vi "EnQ Vacuum State.vi"(6 "Raw Pressure":dbl=nan, 7 "d/dt":dbl, 8 "error in (no error)":errorcluster, 9 "Pressure":dbl=nan, 10 "State":T1, 11 "cRIO Vacuum in":refnum<class "cRIO Vacuum.lvclass">) -> (0 "error out":errorcluster, 1 "overflow?":bool, 2 "Overflow State":T1, 3 "cRIO Vacuum out":refnum<class "cRIO Vacuum.lvclass">, 4 "Overflow Pressure":dbl, 5 "Overflow Raw Pressure":dbl)   [LabVIEW 2015, in "cRIO-Carbondioxide.lvlib" / "CO2-Actor.lvlib" / "cRIO Vacuum.lvclass"]
uses:
  cRIO Vacuum.lvclass
  Controls/Vacuum State Enumerator.ctl
  Controls/Vacuum State Cluster.ctl
  cRIO Vacuum.lvclass/cRIO Vacuum.ctl
panel:
  out "Overflow d/dt":dbl
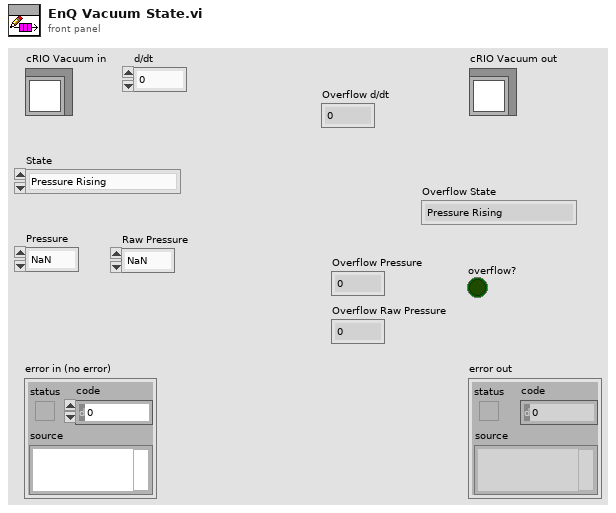
[diagram p1: front panel]
types:
  T1 = typedef "Vacuum State Enumerator.ctl" = enum16{"Pressure Rising", "Plateau", "Pressure Dropping", "Valley", "Low Valley", "Leak", "Unknown"}
  T2 = typedef "Vacuum State Cluster.ctl" = cluster{"Vacuum State":T1, "Pressure":dbl, "Raw Pressure":dbl, "d/dt":dbl}
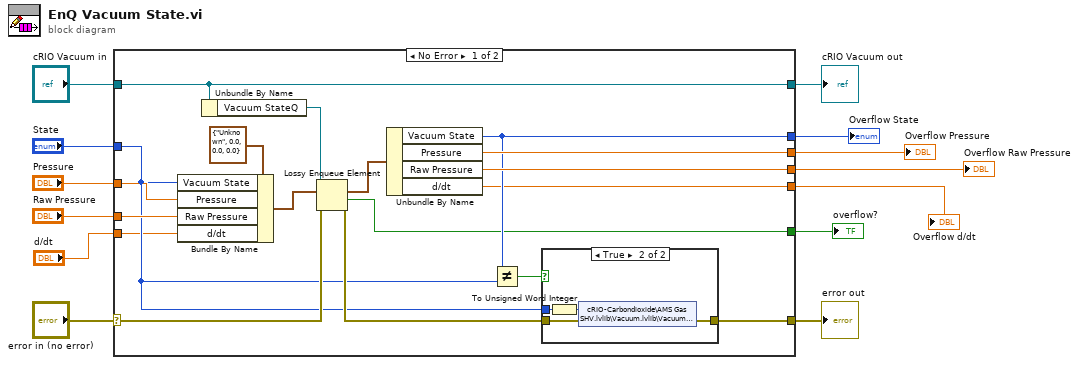
[diagram p0: block diagram]
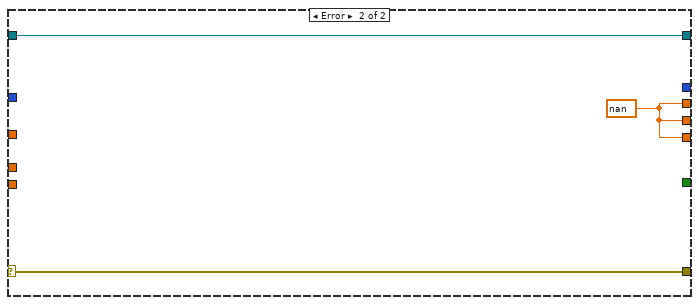
[diagram p3: hidden frame]
diagram:
  n1 = case shown="No Error" "error in (no error)" {
    selector: "error in (no error)" -> [w30 w38]
    tunnel: [w22 w38] -> w12
    tunnel: [w31 w39] -> w10
    tunnel: "cRIO Vacuum in" -> [w31 w39]
    tunnel: "State" -> [w20 _]
    tunnel: [w24 _] -> w8
    tunnel: [w15 _] -> w7
    tunnel: "Pressure" -> [w26 _]
    tunnel: [w28 w37] -> w5
    tunnel: "Raw Pressure" -> [w27 _]
    tunnel: [w25 w37] -> w3
    tunnel: "d/dt" -> [w16 _]
    tunnel: [w14 w37] -> w1
    frame No Error {
      n2 = Bundle By Name(cluster=T2 {"Vacuum State"=enum."Unknown", "Pressure"=0.0, "Raw Pressure"=0.0, "d/dt"=0.0} ("element"), "Vacuum State"=w20, "Pressure"=w26, "Raw Pressure"=w27, "d/dt"=w16) -> (w17:T2)
      n3 = Unbundle By Name(w31) -> ("Vacuum StateQ"=w19:refnum<queue>)
      n4 = Lossy Enqueue Element(queue=w19, element=w17, error in (no error)=w30) -> (overflow element=w29:T2, overflow?=w15:bool, error out=w23:errorcluster)  [unwired: 1 out]
      n5 = Unbundle By Name(w29) -> ("Vacuum State"=w24:T1, "Pressure"=w28:dbl, "Raw Pressure"=w25:dbl, "d/dt"=w14:dbl)
      n6 = Not Equal?(x=w24, y=w20) -> (x != y?=w21:bool)
      n7 = case shown="True" w21 {
        tunnel: w23 -> [w32 w36]
        tunnel: [w32 w35] -> w22
        tunnel: w20 -> [_ w34]
        frame False {
        }
        frame True {
          n8 = To Unsigned Word Integer(number=w34) -> (unsigned 16bit integer=w33:u16)
          n9 = shared-variable "cRIO-Carbondioxide\\AMS Gas SHV.lvlib\\Vacuum.lvlib\\Vacuum State"(w33, error in=w36) -> (error out=w35:errorcluster)
        }
      }
    }
    frame Error {
      w37 = nan ("Pressure")
    }
  }
  "error out" <- w12
  "cRIO Vacuum out" <- w10
  "Overflow State" <- w8
  "overflow?" <- w7
  "Overflow Pressure" <- w5
  "Overflow Raw Pressure" <- w3
  "Overflow d/dt" <- w1
